vi "Tokenizer.vi"(1 "Input String":string) -> (0 "Tokenized Array":string[](array[string]))   [LabVIEW 2012]
uses:
  <vilib>/regexp/Match Regular Expression.xnode
panel:
  out "Next String Start":dbl
  out "Debug Display":string caption="{Before} {Matched} {After} {... submatches ...}"
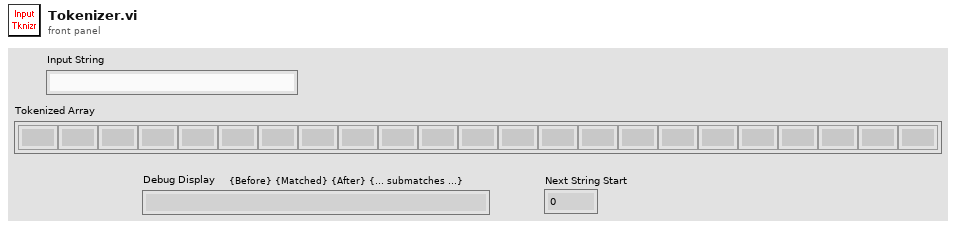
[diagram p1: front panel]
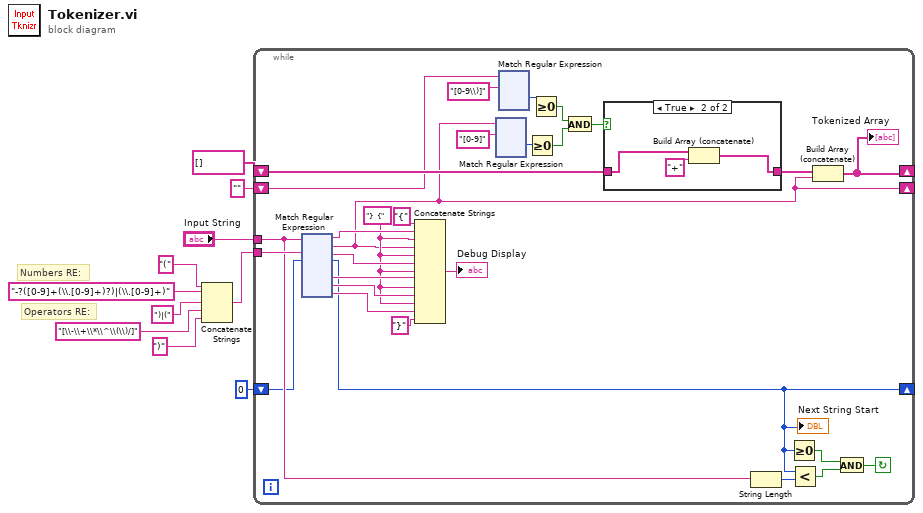
[diagram p0: block diagram]
diagram:
  # "Operators RE:"
  # "Numbers RE:"
  n1 = Concatenate Strings("(", "-?([0-9]+(\\.[0-9]+)?)|(\\.[0-9]+)", ")|(", "[\\-\\+\\*\\^\\(\\)/]", ")") -> (w4:string)
  n2 = while {
    shift-right: [w22] -> _
    shift-left: string[] [] -> [w26]
    shift-right: [w11] -> _
    shift-left: 0 ("offset (0)") -> [w16]
    tunnel: w4 -> [w36]
    shift-right: [w24] -> _
    shift-left: "" ("whole match") -> [w23]
    tunnel: "Input String" -> [w17]
    stop <- w15 continue-if-true
    w32 = "}  {"
    n3 = xnode "Match Regular Expression"("input string"=w17, "regular expression"=w36, "offset (0)"=w16) -> ("before match"=w33:string, "whole match"=w24:string, "after match"=w39:string, "offset past match"=w11:i32, "submatch 1"=w38:string, "submatch 2"=w37:string, "submatch 3"=w35:string)  [unwired: 3 in, 1 out]
    "Next String Start" <- w11
    n4 = Concatenate Strings("{", w33, w32, w24, w32, w39, w32, w38, w32, w37, w32, w35, "}" ("string")) -> (→"Debug Display":string)
    n5 = xnode "Match Regular Expression"("input string"=w24, "regular expression"="[0-9]") -> ("offset past match"=w21:i32)  [unwired: 4 in, 4 out]
    n6 = xnode "Match Regular Expression"("input string"=w23, "regular expression"="[0-9\\)]") -> ("offset past match"=w20:i32)  [unwired: 4 in, 4 out]
    n7 = Greater Or Equal To 0?(x=w21) -> (x >= 0?=w18:bool)
    n8 = Greater Or Equal To 0?(x=w20) -> (x >= 0?=w19:bool)
    n9 = And(x=w19, y=w18) -> (x .and. y?=w27:bool)
    n10 = case shown="True" w27 {
      tunnel: w26 -> [w262 w264]
      tunnel: [w262 w263] -> w25
      frame False {
      }
      frame True {
        n11 = Build Array (concatenate)(w264, "+") -> (w263:string[])
      }
    }
    n12 = String Length(string=w17) -> (length=w12:i32)
    n13 = Greater Or Equal To 0?(x=w11) -> (x >= 0?=w14:bool)
    n14 = Less?(x=w11, y=w12) -> (x < y?=w13:bool)
    n15 = Build Array (concatenate)(w25, w24) -> (w22:string[])
    "Tokenized Array" <- w22
    n16 = And(x=w14, y=w13) -> (x .and. y?=w15:bool)
  }
